vi "Read SystemConfigurationChange.vi"(8 "error in (no error)":errorcluster, 11 "SystemConfiguration in":refnum<class "SystemConfiguration.lvclass">) -> (0 "error out":errorcluster, 2 "SystemConfigurationChange":string, 3 "SystemConfiguration out":refnum<class "SystemConfiguration.lvclass">)   [LabVIEW 2019, in "SystemSetup.lvlib" / "SystemConfiguration.lvclass"]
uses:
  SystemConfiguration.lvclass
  SystemConfiguration.lvclass/SystemConfiguration.ctl
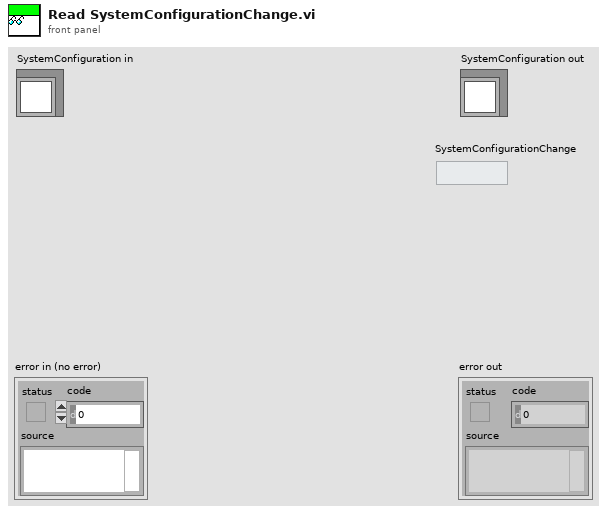
[diagram p1: front panel]
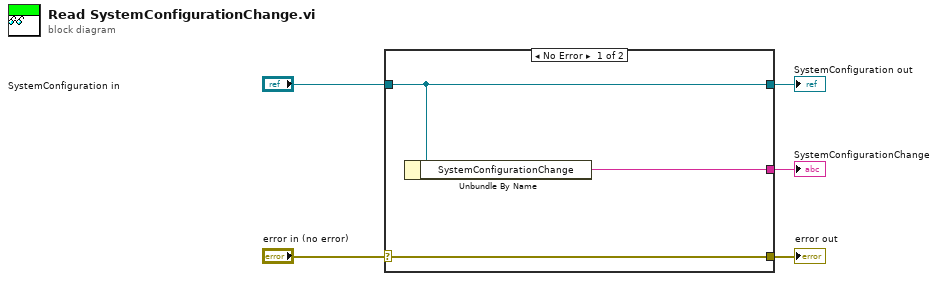
[diagram p0: block diagram]
diagram:
  n1 = case shown="No Error" "error in (no error)" {
    selector: "error in (no error)" -> [w8 w9]
    tunnel: [w8 w9] -> w4
    tunnel: [w7 w10] -> w2
    tunnel: "SystemConfiguration in" -> [w7 w10]
    tunnel: [w6 _] -> w1
    frame No Error {
      n2 = Unbundle By Name(w7) -> ("SystemConfigurationChange"=w6:string)
    }
    frame Error {
    }
  }
  "error out" <- w4
  "SystemConfiguration out" <- w2
  "SystemConfigurationChange" <- w1
